vi "read_photosensor.vi"(7 "error in":errorcluster, 9 "number of samples":i32=-1, 10 "task/channels in":refnum<k21>) -> (0 "error out":errorcluster, 3 "Avg Voltage":dbl=1000.0 format="%0.2f")   [LabVIEW 2018]
doc: "This example demonstrates how to continuously acquire buffered voltage measurements using a DAQmx device.\n\nFor instructions on how to connect your signals to the DAQ device, refer to your device documentation."
uses:
  SupportVIs/DAQmx Read (Analog 1D Wfm NChan NSamp).vi
  SupportVIs/DAQmx Fill In Error Info.vi
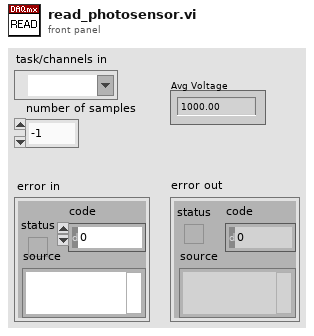
[diagram p1: front panel]
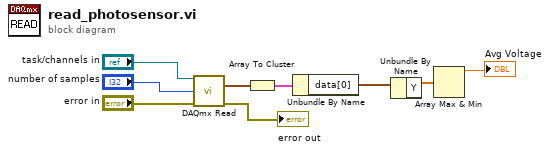
[diagram p0: block diagram]
diagram:
  n1 = call-poly "DAQmx Read.vi"("task/channels in"="task/channels in", "number of samples per channel"="number of samples", "error in"="error in") -> ("data"=w9:waveform(dbl)[], "error out"=→"error out":errorcluster)  [unwired: 10 in, 1 out]
  n2 = Array To Cluster(array=w9) -> (cluster=w8:cluster{"data[0]":waveform(dbl)})
  n3 = Unbundle By Name(w8) -> ("data[0]"=w6:waveform(dbl))
  n4 = Unbundle By Name(w6) -> ("Y"=w7:dbl[])
  n5 = Array Max & Min(array=w7) -> (max value=→"Avg Voltage":dbl)  [unwired: 3 out]
